vi "change password sub.vi"(7 "Array in":T1(array[ring]), 8 "error in (no error)":errorcluster, 9 "RingText.Text":string, 10 "Lock State":T2(ring)=enum."Password-protected", 11 "Path":path) -> (0 "error out":errorcluster, 3 "Array out":T1(array[ring]))   [LabVIEW 2013]
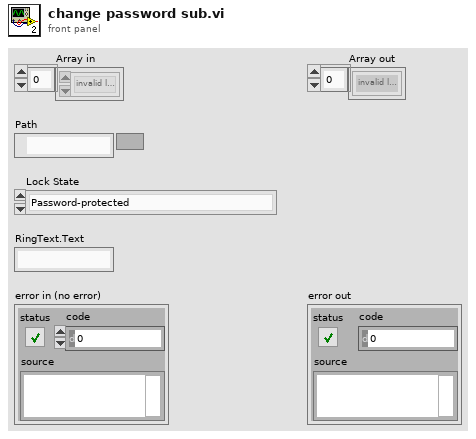
[diagram p1: front panel]
types:
  T1 = enum32{"invalid lock state", "Not Locked", "Locked (No Password)", "Password-protected"}[]
  T2 = enum32{"invalid lock state", "Not Locked", "Locked (No Password)", "Password-protected"}
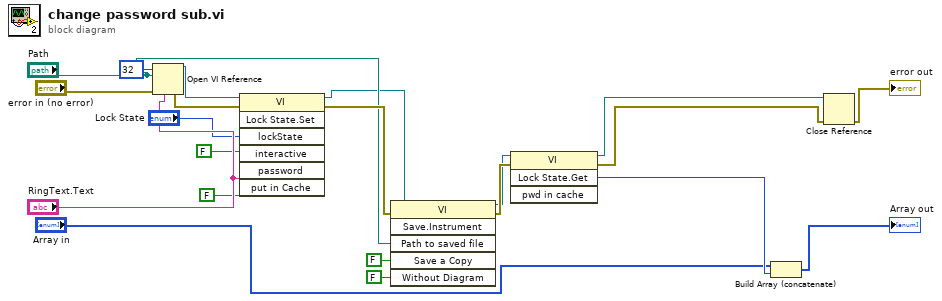
[diagram p0: block diagram]
diagram:
  n1 = Open VI Reference(vi path="Path", options=32, password ("")="RingText.Text", error in (no error)="error in (no error)") -> (vi reference=w1:refnum<vi>, error out=w5:errorcluster)  [unwired: 2 in]
  n2 = invoke class="VI" method="Lock State.Set"(reference=w1, error in=w5, "lockState"="Lock State", "interactive"=FALSE ("Interactive"), "password"="RingText.Text", "put in Cache"=FALSE ("Put in Cache")) -> (reference out=w8:refnum<vi>, error out=w17:errorcluster)  [unwired: 1 in, 5 out]
  n3 = invoke class="VI" method="Save.Instrument"(reference=w8, error in=w17, "Path to saved file"="Path", "Save a Copy"=FALSE, "Without Diagram"=FALSE) -> (reference out=w9:refnum<vi>, error out=w18:errorcluster)  [unwired: 1 in, 4 out]
  n4 = invoke class="VI" method="Lock State.Get"(reference=w9, error in=w18) -> (reference out=w6:refnum<vi>, error out=w7:errorcluster, "Get Lock State"=w14:T2)  [unwired: 2 in, 1 out]
  n5 = Build Array (concatenate)("Array in", w14) -> (→"Array out":T1)
  n6 = Close Reference(reference=w6, error in (no error)=w7) -> (error out=→"error out":errorcluster)
